vi "WPI_CANJaguar_ConfigEncoderCodesPerRev.vi"(8 "error in (no error)":errorcluster, 10 "Encoder Codes Per Rev":u16=64, 11 "CAN Jaguar Ref":T1={"DeviceStatus"={"status"=FALSE, "code"=0, "source"=""}, "Type"=enum."PWM", "PWM"={"PWM Channel"=enum."PWM 1", "DeadBand"={"Name"="", "maxPositivePwm"=0, "minPositivePwm"=0, "centerPwm"=0, "maxNegativePwm"=0, "minNegativePwm"=0, "angularRange"=0}}, "CAN"={"Device Number"=0, "SetOutput VI Ref"=variant(enum8{"Percent VBus", "Current", "Speed", "Position", "Voltage"} enum."Percent VBus"), "GetOutput VI Ref"=variant(refnum<k1> refnum), "Enable VI Ref"=variant(dbl 12.0), "Disable VI Ref"=variant(enum8{"Percent VBus", "Speed", "Position", "Slave", "Unchanged / Invalid", "Voltage Compensation", "Current", "Motion Profile"} enum."Percent VBus"), "Data"=variant}, "Invert"=FALSE}) -> (0 "error out":errorcluster, 3 "CAN Jaguar Ref":T1={"DeviceStatus"={"status"=FALSE, "code"=0, "source"=""}, "Type"=enum."PWM", "PWM"={"PWM Channel"=enum."PWM 1", "DeadBand"={"Name"="", "maxPositivePwm"=0, "minPositivePwm"=0, "centerPwm"=0, "maxNegativePwm"=0, "minNegativePwm"=0, "angularRange"=0}}, "CAN"={"Device Number"=0, "SetOutput VI Ref"=variant(enum8{"Percent VBus", "Current", "Speed", "Position", "Voltage"} enum."Percent VBus"), "GetOutput VI Ref"=variant(refnum<k1> refnum), "Enable VI Ref"=variant(dbl 12.0), "Disable VI Ref"=variant(enum8{"Percent VBus", "Speed", "Position", "Slave", "Unchanged / Invalid", "Voltage Compensation", "Current", "Motion Profile"} enum."Percent VBus"), "Data"=variant}, "Invert"=FALSE})   [LabVIEW 2016]
doc: "Configures the number codes in one revolution of the encoder. This is used in scaling the value in <B>Set Output</B> and <B>Get Output</B> when in <B>Position</B> or <B>Speed</B> control mode as well as <B>Get Status::Position</B> and <B>Get Status::Speed</B>."
uses:
  <vilib>/Rock Robotics/WPI/MotorControl/WPI_MotorControlDeviceRef.ctl
  <vilib>/Rock Robotics/WPI/MotorControl/WPI_MotorControlType.ctl
  <vilib>/Rock Robotics/SystemInterfaces/DIO/FPGA_DIOPWMChannel.ctl
  <vilib>/Rock Robotics/WPI/PWM/WPI_PWMDeadband.ctl
  <vilib>/Rock Robotics/WPI/ThirdParty/CanMotor/CAN Jaguar/SubVIs/WPI_CAN_MotorMessageIDs.ctl
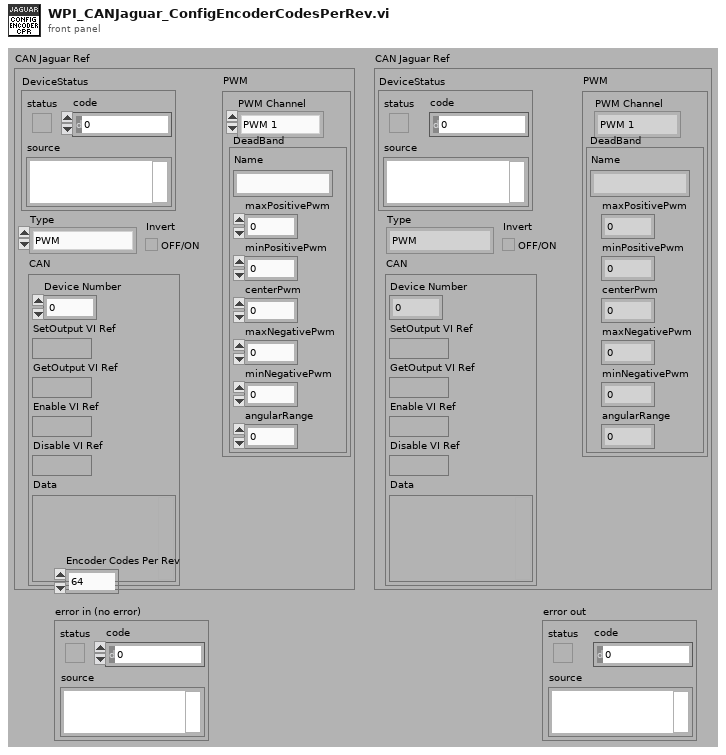
[diagram p1: front panel]
types:
  T1 = typedef "WPI_MotorControlDeviceRef.ctl" = cluster{"DeviceStatus":errorcluster, "Type":T2, "PWM":cluster{"PWM Channel":T3, "DeadBand":T4}, "CAN":cluster{"Device Number":u8, "SetOutput VI Ref":variant, "GetOutput VI Ref":variant, "Enable VI Ref":variant, "Disable VI Ref":variant, "Data":variant}, "Invert":bool}
  T2 = typedef "WPI_MotorControlType.ctl" = enum16{"PWM", "CAN"}
  T3 = typedef "FPGA_DIOPWMChannel.ctl" = enum8{"PWM 0", "PWM 1", "PWM 2", "PWM 3", "PWM 4", "PWM 5", "PWM 6", "PWM 7", "PWM 8", "PWM 9", "PWM MXP 0", "PWM MXP 1", "PWM MXP 2", "PWM MXP 3", "PWM MXP 4", "PWM MXP 5", "PWM MXP 6", "PWM MXP 7", "PWM MXP 8", "PWM MXP 9", "Invalid"}
  T4 = typedef "WPI_PWMDeadband.ctl" = cluster{"Name":string, "maxPositivePwm":i32, "minPositivePwm":i32, "centerPwm":i32, "maxNegativePwm":i32, "minNegativePwm":i32, "angularRange":u16}
  T5 = enum16{"big-endian, network order", "native, host order", "little-endian"}
  T6 = typedef "WPI_CAN_MotorMessageIDs.ctl" = u32
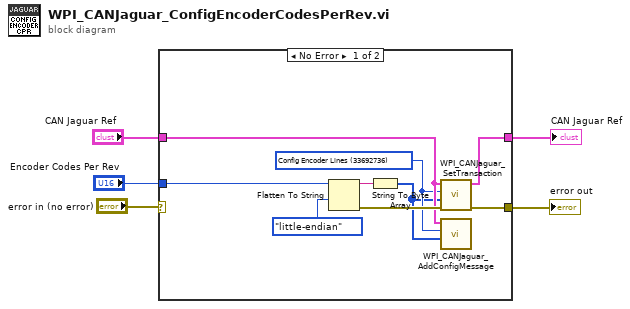
[diagram p0: block diagram]
diagram:
  n1 = case shown="No Error" "error in (no error)" {
    selector: "error in (no error)" -> [_ w16]
    tunnel: [w11 w16] -> w5
    tunnel: [w9 w15] -> w3
    tunnel: "CAN Jaguar Ref" -> [w8 w15]
    tunnel: "Encoder Codes Per Rev" -> [w14 _]
    frame No Error {
      w7 = T6 33692736 items=["Volt Enable"=33685504, "Volt Disable"=33685568, "Volt Set"=33685632, "Volt Set Ramp"=33685696, "Speed Enable"=33686528, "Speed Disable"=33686592, "Speed Set"=33686656, "Speed P"=33686720, "Speed I"=33686784, "Speed D"=33686848, "Speed Ref"=33686912, "Volt Comp Enable"=33687552, "Volt Comp Disable"=33687616, "Volt Comp Set"=33687680, "Volt Comp In Ramp"=33687744, "Volt Comp Comp Ramp"=33687808, "Position Enable"=33688576, "Position Disable"=33688640, "Position Set"=33688704, "Position P"=33688768, "Position I"=33688832, "Position D"=33688896, "Position Ref"=33688960, "Current Enable"=33689600, "Current Disable"=33689664, "Current Set"=33689728, "Current P"=33689792, "Current I"=33689856, "Current D"=33689920, "Status Percent VBus"=33690624, "Status VBus"=33690688, "Status Current"=33690752, "Status Temp"=33690816, "Status Position"=33690880, "Status Speed"=33690944, "Status Limit"=33691008, "Status Fault"=33691072, "Status Power"=33691136, "Status Control Mode"=33691200, "Status VOut"=33691264, "Config Num Brushes"=33692672, "Config Encoder Lines"=33692736, "Config Pot Turns"=33692800, "Config Brake Coast"=33692864, "Config Limit Mode"=33692928, "Config Limit Fwd"=33692992, "Config Limit Rev"=33693056, "Config Max VOut"=33693120, "Config Fault Time"=33693184, "Motor Ack"=33693696] ("CAN Motor Message IDs")
      n2 = Flatten To String(anything=w14, byte order (0:big-endian, network order)=T5."little-endian") -> (data string=w12:string, error out=w10:errorcluster)  [unwired: 1 in, 2 out]
      n3 = String To Byte Array(string=w12) -> (unsigned byte array=w6:u8[])
      n4 = call <vilib>:"WPI_CANJaguar_SetTransaction.vi"("error in"=w10, "Data"=w6, "Message ID"=w7, "CAN Jaguar Ref"=w8) -> ("error out"=w11:errorcluster, "CAN Jaguar Ref Out"=w9:T1)  [unwired: 6 out]
      n5 = call <vilib>:"WPI_CANJaguar_AddConfigMessage.vi"("Data"=w6, "Message ID"=w7, "CAN Jaguar Ref"=w8) -> ()  [unwired: 9 in]
    }
    frame Error {
    }
  }
  "CAN Jaguar Ref" <- w3
  "error out" <- w5
